vi "InputAndTargetOutput.vi"(7 "Arduino Digital Outputs":u8[](array[numeric])=[2, 3, 4, 5, 6], 8 "Decimal Input into\nLogic Block":u8=1, 9 "Designated Garbage Pin":i32, 10 "Error In":errorcluster, 11 "LINX Resource Input":T1) -> (0 "Target Output":u32, 1 "Arduino Digital Outputs 2":u8[](array[numeric])=[2, 3, 4, 5, 6], 2 "Error Out":errorcluster, 3 "LINX Resource Output":T1, 4 "Binary Inputs into\nLogic Block":bool[](array[boolean]), 5 "Numerical\nInput Troubleshoot":u32)   [LabVIEW 2018]
uses:
  <vilib>/MakerHub/LINX/Private/Type Defs/LINX Ref.ctl
  <vilib>/MakerHub/LINX/Private/Type Defs/Platform.ctl
  <vilib>/MakerHub/LINX/Private/Type Defs/Interface.ctl
  <vilib>/MakerHub/LINX/Private/Device/Type Defs/LINX Device Config.ctl
  <vilib>/MakerHub/LINX/Private/Device/Type Defs/TCP Config.ctl
  <vilib>/MakerHub/LINX/Private/Device/Type Defs/Channels.ctl
  <vilib>/MakerHub/LINX/Public/Peripherals/Digital/Digital Write N Chans.vi
  <vilib>/MakerHub/LINX/Private/Local IO/LinxDigitalWrite.vi
  <vilib>/MakerHub/LINX/Public/Utilities/Check Channel.vi
  <vilib>/MakerHub/LINX/Private/Utilties/Generate Error.vi
  <vilib>/MakerHub/LINX/LMH-LINX.lvlib
  <vilib>/MakerHub/LINX/Private/Device/Device.lvlib
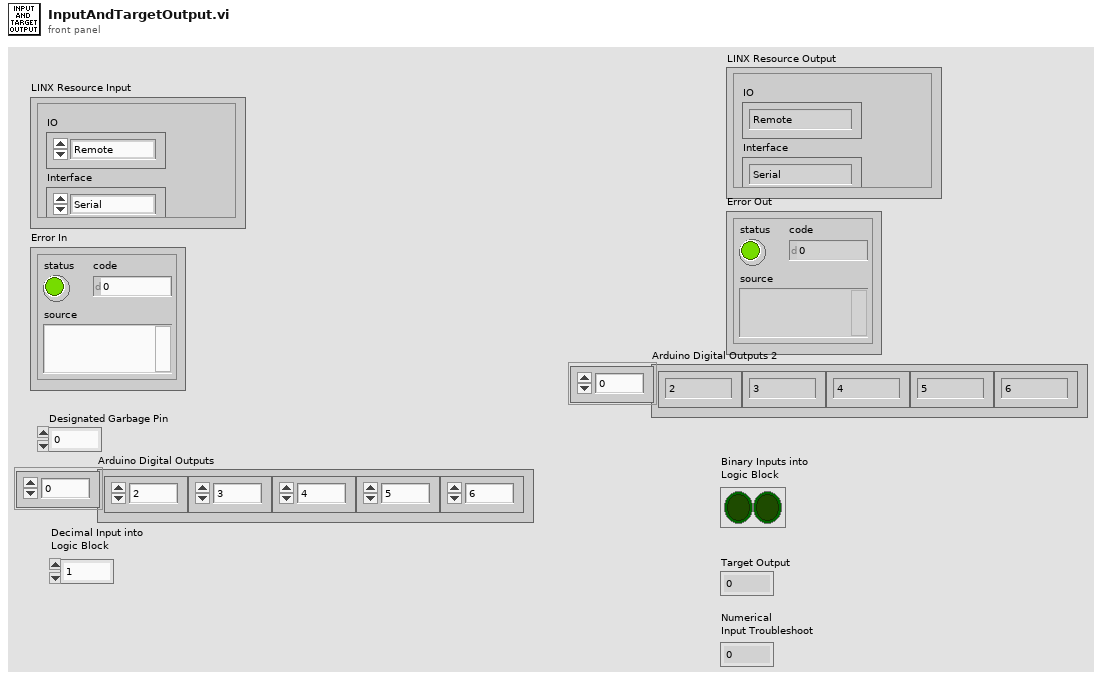
[diagram p1: front panel]
types:
  T1 = typedef "LMH-LINX.lvlib/LINX Ref.ctl" = cluster{"IO":T2, "Interface":T3, "LINX Device Config":T4}
  T2 = typedef "LMH-LINX.lvlib/Platform.ctl" = enum16{"Remote", "Local"}
  T3 = typedef "LMH-LINX.lvlib/Interface.ctl" = enum16{"Serial", "TCP"}
  T4 = typedef "LMH-LINX.lvlib/Device.lvlib/LINX Device Config.ctl" = cluster{"Interface":T3, "COM Port":refnum<visa-resource-name>, "TCP Configuration":T5, "Device Family":u8, "Device ID":u8, "Device Name":string, "TCP Ref":refnum<k5>, "Channels":T6}
  T5 = typedef "LMH-LINX.lvlib/Device.lvlib/TCP Config.ctl" = cluster{"IP Address":string, "Port":u16}
  T6 = typedef "LMH-LINX.lvlib/Channels.ctl" = cluster{"DI":u8[], "DO":u8[], "AI":u8[], "AO":u8[], "PWM":u8[], "QE":u8[], "UART":u8[], "I2C 2":u8[], "SPI":u8[], "CAN":u8[], "Servo":u8[], "AI Ref (V)":dbl, "AI Resolution (Bits)":u8, "AO Ref (V)":dbl, "AO Resolution (Bits)":u8}
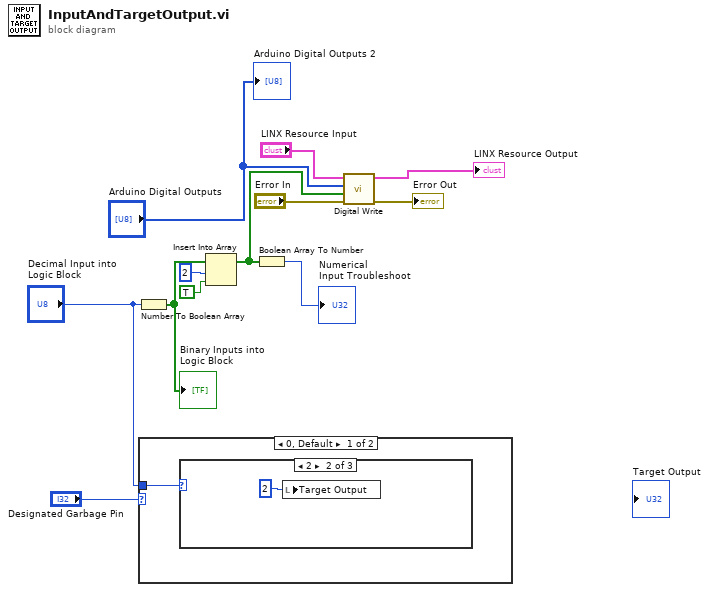
[diagram p0: block diagram]
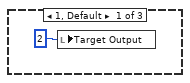
[diagram p2: hidden frame]
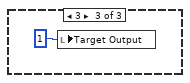
[diagram p3: hidden frame]
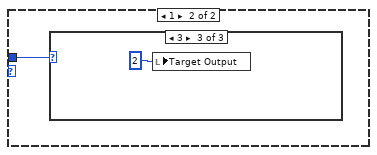
[diagram p4: hidden frame]
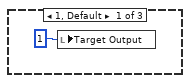
[diagram p5: hidden frame]
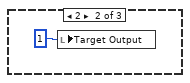
[diagram p6: hidden frame]
diagram:
  n1 = Number To Boolean Array(number="Decimal Input into\nLogic Block") -> (Boolean array=w10:bool[])
  "Binary Inputs into\nLogic Block" <- w10
  n2 = case shown="0, Default" "Designated Garbage Pin" {
    tunnel: "Decimal Input into\nLogic Block" -> [w13 w17]
    frame 0, Default {
      n3 = case shown="2" w13 {
        frame 1, Default {
          n4 = local write "Target Output"(2) -> ()
        }
        frame 2 {
          n5 = local write "Target Output"(u32 2 ("Target Output")) -> ()
        }
        frame 3 {
          n6 = local write "Target Output"(u32 1 ("Target Output")) -> ()
        }
      }
    }
    frame 1 {
      n7 = case shown="3" w17 {
        frame 1, Default {
          n8 = local write "Target Output"(1) -> ()
        }
        frame 2 {
          n9 = local write "Target Output"(u32 1 ("Target Output")) -> ()
        }
        frame 3 {
          n10 = local write "Target Output"(u32 2 ("Target Output")) -> ()
        }
      }
    }
  }
  n11 = Insert Into Array(array=w10, index=2, new element=TRUE ("new element/subarray")) -> (w8:bool[])
  n12 = Boolean Array To Number(Boolean array=w8) -> (number=→"Numerical\nInput Troubleshoot":u32)
  n13 = call-poly <vilib>:"Digital Write.vi"("Error In"="Error In", "Values"=w8, "DO Channels"="Arduino Digital Outputs", "LINX Resource"="LINX Resource Input") -> ("Error Out"=→"Error Out":errorcluster, "LINX Resource"=→"LINX Resource Output":T1)  [unwired: 6 in]
  "Arduino Digital Outputs 2" <- "Arduino Digital Outputs"
